vi "Camera.vi"(7 "Machine Vision":T3, 8 "error in (no error)":errorcluster, 10 "Stop":bool, 11 "Camera in":refnum<class "Camera.lvclass">) -> (0 "error out":errorcluster, 1 "Camera":dbl[](array[numeric]), 2 "Image":T2(plugin-control), 3 "Camera out":refnum<class "Camera.lvclass">, 4 "Image Out":T2(plugin-control), 5 "Numeric":dbl, 6 "camera R":dbl)   [LabVIEW 2016, in "Camera.lvclass"]
uses:
  Camera.lvclass
  Machine Vision.ctl
  <vilib>/Analysis/coordinate.llb/2D Cartesian Coordinate Rotation (Scalar).vi
  <vilib>/Analysis/NI_AALPro.lvlib
panel:
  out "Fitted Circle (Find Circular Edge 1) 2":T1 {"Average SNR (dB)" format="%.2f"; "Average Strength" format="%.2f"; "Roundness (Real-World)" format="%.2f"; "Radius (Real-World)" format="%.2f"; "Center (Real-World)"."Y" format="%.2f"; "Center (Real-World)"."X" format="%.2f"; "Radius (Pixels)" format="%.2f"; "Center (Pixels)"."Y" format="%.2f"; "Center (Pixels)"."X" format="%.2f"}
  out "Fitted Circle (Find Circular Edge 1)":T1 {"Average SNR (dB)" format="%.2f"; "Average Strength" format="%.2f"; "Roundness (Real-World)" format="%.2f"; "Radius (Real-World)" format="%.2f"; "Center (Real-World)"."Y" format="%.2f"; "Center (Real-World)"."X" format="%.2f"; "Radius (Pixels)" format="%.2f"; "Center (Pixels)"."Y" format="%.2f"; "Center (Pixels)"."X" format="%.2f"}
  out "subarray 2":sgl[](array[numeric])
  out "subarray":sgl[](array[numeric])
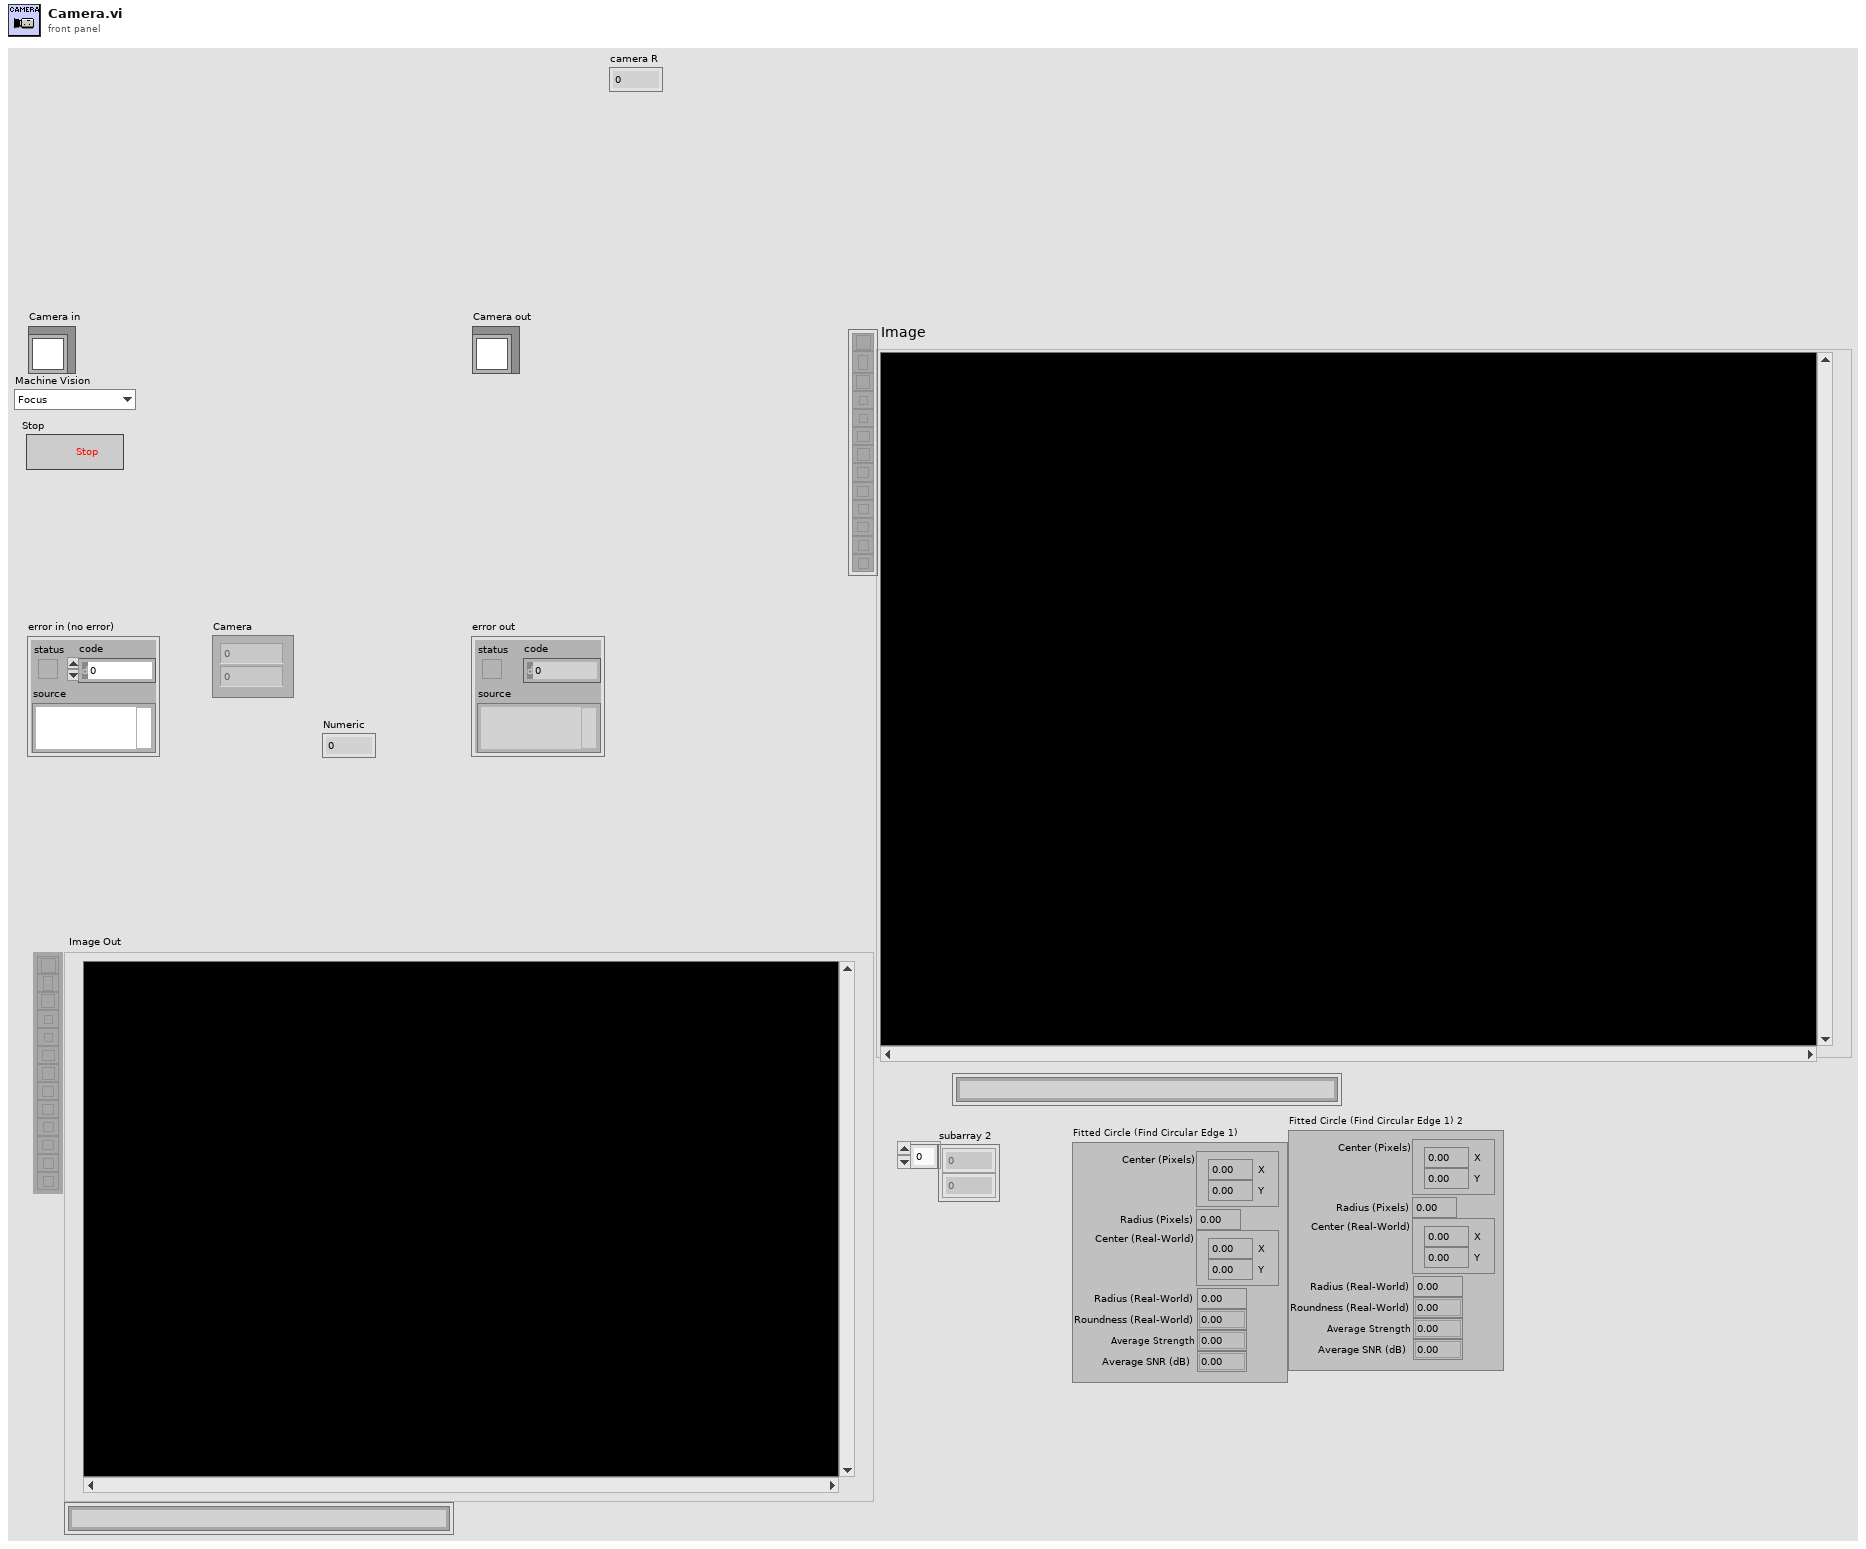
[diagram p1: front panel]
types:
  T1 = cluster{"Center (Pixels)":cluster{"X":sgl, "Y":sgl}, "Radius (Pixels)":dbl, "Center (Real-World)":cluster{"X":sgl, "Y":sgl}, "Radius (Real-World)":dbl, "Roundness (Real-World)":dbl, "Average Strength":dbl, "Average SNR (dB)":dbl}
  T2 = typedef "IMAQ Image.ctl" = refnum<image>
  T3 = typedef "Camera.lvclass/Machine Vision.ctl" = enum16{"Focus", "chip cross", "LargeCircle", "None", "INTT HDI Mark", "INTT Sensor Cross", "INTT Chip Corner", "HPK Silicon", "circle"}
  T4 = typedef "IMAQ GM Match Report.ctl" = cluster{"Position":cluster{"x":sgl, "y":sgl}, "Angle":sgl, "Scale":sgl, "Score":sgl, "Bounding Box":cluster{"x":sgl, "y":sgl}[], "Contrast Reversed":bool, "Occlusion %":sgl, "Template Target Curve Score":sgl, "Target Template Curve Score":sgl, "Correlation Score":sgl}
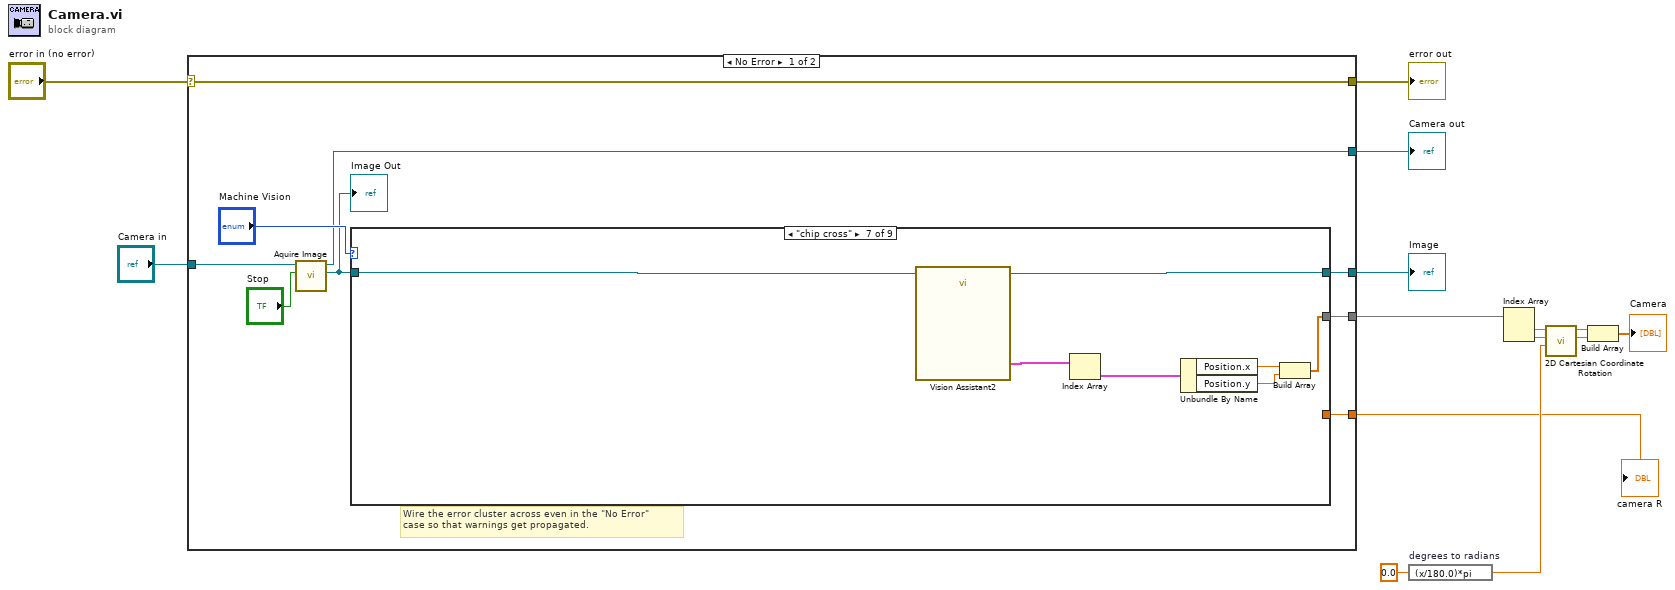
[diagram p0: block diagram]
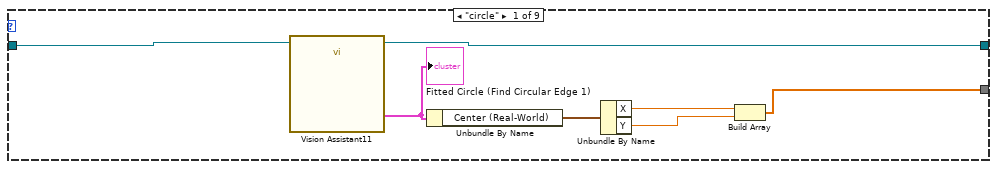
[diagram p2: hidden frame]
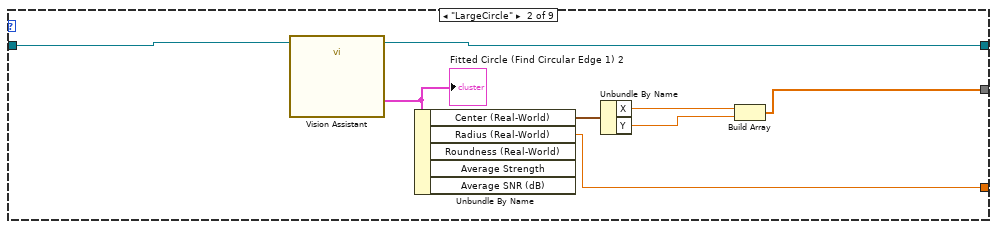
[diagram p3: hidden frame]
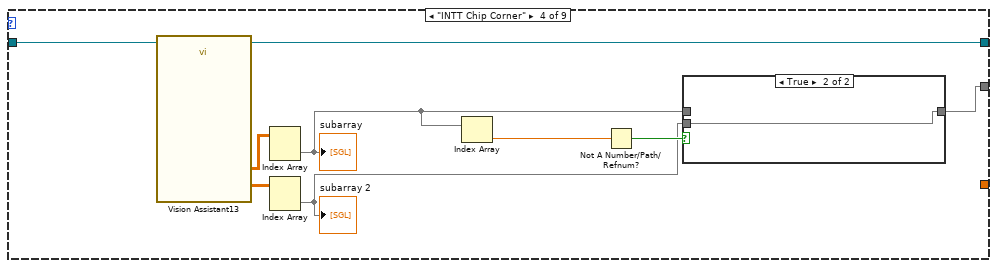
[diagram p5: hidden frame]
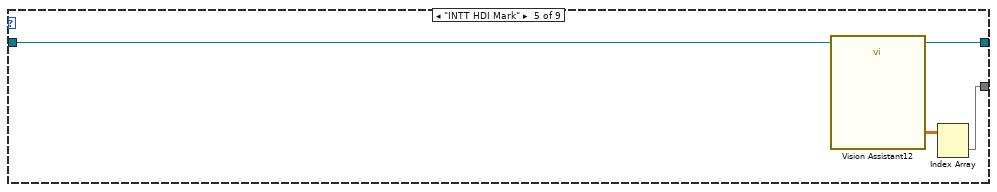
[diagram p7: hidden frame]
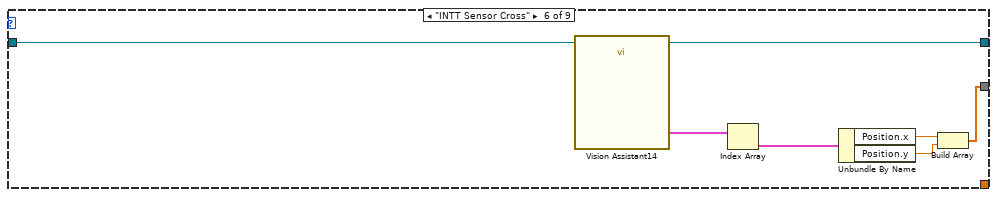
[diagram p8: hidden frame]
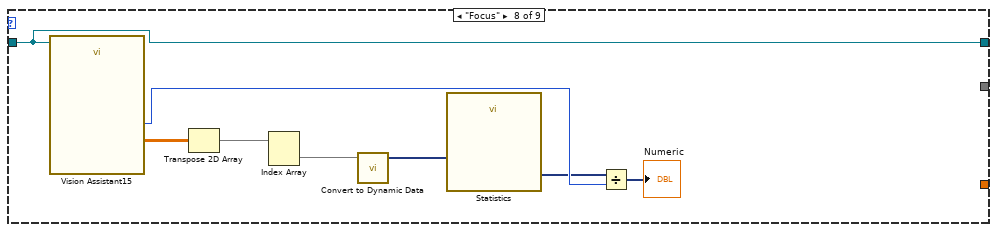
[diagram p9: hidden frame]
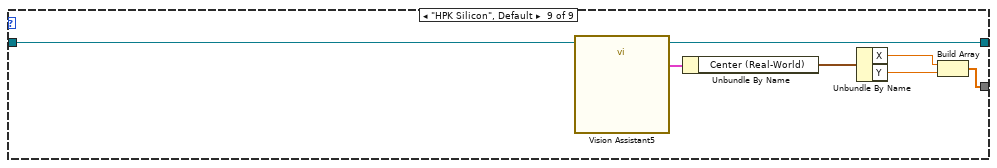
[diagram p10: hidden frame]
diagram:
  n1 = case shown="No Error" "error in (no error)" {
    selector: "error in (no error)" -> [w23 w85]
    tunnel: [w23 w85] -> w13
    tunnel: [w19 w84] -> w12
    tunnel: "Camera in" -> [w20 w84]
    tunnel: [w18 _] -> w7
    tunnel: [w17 _] -> w10
    tunnel: [w15 _] -> w1
    frame No Error {
      # "Wire the error cluster across even in the \"No Error\"\ncase so that warnings get propagated."
      n2 = call-dynamic "Aquire Image.vi"("Stop"="Stop", "Camera in"=w20) -> ("Image Out"=w16:T2, "Camera out"=w19:refnum<class "Camera.lvclass">)  [unwired: 7 in, 1 out]
      "Image Out" <- w16
      n3 = case shown="\"chip cross\"" "Machine Vision" {
        tunnel: [w24 w33 _ w40 w52 w57 w64 _ w78] -> w18
        tunnel: [w25 w34 w39 w43 w53 w56 w63 w75 w80] -> w17
        tunnel: w16 -> [w27 w35 w39 w42 w54 w55 w62 w75 w79]
        tunnel: [_ w31 _ _ _ _ _ _ _] -> w15
        frame "circle" {
          n4 = call "Vision Assistant11"("Image In"=w27) -> ("Image Out"=w25:T2, "Fitted Circle (Find Circular Edge 1)"=w26:T1)  [unwired: 24 in, 1 out]
          "Fitted Circle (Find Circular Edge 1)" <- w26
          n5 = Unbundle By Name(w26) -> ("Center (Real-World)"=w30:cluster{"X":sgl, "Y":sgl})
          n6 = Unbundle By Name(w30) -> ("X"=w29:sgl, "Y"=w28:sgl)
          n7 = Build Array(w29, w28) -> (w24:sgl[])
        }
        frame "LargeCircle" {
          n8 = call "Vision Assistant"("Image In"=w35) -> ("Image Out"=w34:T2, "Fitted Circle (Find Circular Edge 1)"=w32:T1)  [unwired: 24 in, 1 out]
          "Fitted Circle (Find Circular Edge 1) 2" <- w32
          n9 = Unbundle By Name(w32) -> ("Center (Real-World)"=w38:cluster{"X":sgl, "Y":sgl}, "Radius (Real-World)"=w31:dbl)  [unwired: 3 out]
          n10 = Unbundle By Name(w38) -> ("X"=w37:sgl, "Y"=w36:sgl)
          n11 = Build Array(w37, w36) -> (w33:sgl[])
        }
        frame "None" {
        }
        frame "INTT Chip Corner" {
          n12 = call "Vision Assistant13"("Image In"=w42) -> ("Image Out"=w43:T2, "Calibrated Results (Caliper 1)"=w48:sgl[][], "Calibrated Results (Caliper 2)"=w45:sgl[][])  [unwired: 17 in, 7 out]
          n13 = Index Array(array=w48) -> (element=w41:sgl[])  [unwired: 2 in]
          "subarray" <- w41
          n14 = Index Array(array=w45) -> (element=w44:sgl[])  [unwired: 2 in]
          "subarray 2" <- w44
          n15 = Index Array(array=w41) -> (element=w47:sgl)  [unwired: 1 in]
          n16 = Not A Number/Path/Refnum?(number/path/refnum=w47) -> (NaN/Path/Refnum?=w46:bool)
          n17 = case shown="True" w46 {
            tunnel: w41 -> [w49 _]
            tunnel: w44 -> [_ w50]
            tunnel: [w49 w50] -> w40
            frame False {
            }
            frame True {
            }
          }
        }
        frame "INTT HDI Mark" {
          n18 = call "Vision Assistant12"("Image In"=w54) -> ("Image Out"=w53:T2, "Calibrated Results (Caliper 5)"=w51:sgl[][])  [unwired: 21 in, 4 out]
          n19 = Index Array(array=w51) -> (element=w52:sgl[])  [unwired: 2 in]
        }
        frame "INTT Sensor Cross" {
          n20 = call "Vision Assistant14"("Image In"=w55) -> ("Image Out"=w56:T2, "Calibrated Matches (Geometric Matching 1)"=w61:T4[])  [unwired: 23 in, 2 out]
          n21 = Index Array(array=w61) -> (element=w60:T4)  [unwired: 1 in]
          n22 = Unbundle By Name(w60) -> ("Position.x"=w59:sgl, "Position.y"=w58:sgl)
          n23 = Build Array(w59, w58) -> (w57:sgl[])
        }
        frame "chip cross" {
          n24 = call "Vision Assistant2"("Image In"=w62) -> ("Image Out"=w63:T2, "Calibrated Matches (Geometric Matching 1)"=w68:T4[])  [unwired: 23 in, 2 out]
          n25 = Index Array(array=w68) -> (element=w67:T4)  [unwired: 1 in]
          n26 = Unbundle By Name(w67) -> ("Position.x"=w66:sgl, "Position.y"=w65:sgl)
          n27 = Build Array(w66, w65) -> (w64:sgl[])
        }
        frame "Focus" {
          n28 = call "Vision Assistant15"("Image In"=w75) -> ("Number of Particles (Particle Analysis 1)"=w76:i32, "Particle Measurements (Pixels) (Particle Analysis 1)"=w74:dbl[][])  [unwired: 22 in, 3 out]
          n29 = Transpose 2D Array(2D array=w74) -> (transposed array=w73:dbl[][])
          n30 = Index Array(array=w73) -> (element=w72:dbl[])  [unwired: 2 in]
          n31 = call "Convert to Dynamic Data"("Array"=w72) -> ("Dynamic Data Type"=w71:dynamicdata)  [unwired: 3 in]
          n32 = call "Statistics"("Signals"=w71) -> ("Summation"=w70:dynamicdata)  [unwired: 25 in, 1 out]
          n33 = Divide(x=w70, y=w76) -> (x/y=→"Numeric":dynamicdata)
        }
        frame "HPK Silicon", Default {
          n34 = call "Vision Assistant5"("Image In"=w79) -> ("Image Out"=w80:T2, "Fitted Circle (Find Circular Edge 1)"=w77:T1)  [unwired: 24 in, 1 out]
          n35 = Unbundle By Name(w77) -> ("Center (Real-World)"=w83:cluster{"X":sgl, "Y":sgl})
          n36 = Unbundle By Name(w83) -> ("X"=w82:sgl, "Y"=w81:sgl)
          n37 = Build Array(w82, w81) -> (w78:sgl[])
        }
      }
    }
    frame Error {
    }
  }
  "error out" <- w13
  "Camera out" <- w12
  "Image" <- w10
  "camera R" <- w1
  n38 = expression code="(x/180.0)*pi" "degrees to radians"(0.0) -> (w4:dbl)
  n39 = Index Array(array=w7) -> (element #1=w6:sgl, element #2=w5:sgl)  [unwired: 2 in]
  n40 = call-poly <vilib>:"2D Cartesian Coordinate Rotation.vi"("theta"=w4, "y"=w5, "x"=w6) -> ("y out"=w2:dbl, "x out"=w8:dbl)  [unwired: 6 in, 1 out]
  n41 = Build Array(w8, w2) -> (→"Camera":dbl[])
